vi "Interpret Admin.vi"(8 "error in (no error)":errorcluster, 11 "VISA resource name":refnum<visa-resource-name>) -> (0 "error out":errorcluster, 2 "Trace Admin":T1 {"X at 0" format="%#_3e"; "Y at 0" format="%#_3e"; "X Resolution" format="%#_3e"; "Y Resolution" format="%#_3e"; "X Offset" format="%#_3e"; "Y Offset" format="%#_3e"; "X Step" items=["1-2-5 Range"=1, "Record Range"=3, "Variable Range"=4]; "Y Step" items=["1-2-5 Range"=1, "1-2-4 Range"=2]; "X Divisions" format="%#_3e"; "Y Divisions" format="%#_3e"; "X Unit" items=["None", "Volt", "Ampere", "Ohm", "Watt", "Farad", "Kelvin", "Seconds", "Hours", "Days", "Hertz", "Degree", "Celsius", "Fahrenheit", "Percentage", "dBm 50 Ohm", "dBm 600 Ohm", "dB Volts", "dB Ampere", "dB Watts", "Volt * Ampere Reactive", "Volt * Ampere"]; "Y Unit" items=["None", "Volt", "Ampere", "Ohm", "Watt", "Farad", "Kelvin", "Seconds", "Hours", "Days", "Hertz", "Degree", "Celsius", "Fahrenheit", "Percentage", "dBm 50 Ohm", "dBm 600 Ohm", "dB Volts", "dB Ampere", "dB Watts", "Volt * Ampere Reactive", "Volt * Ampere"]}, 3 "VISA resource name out":refnum<visa-resource-name>)   [LabVIEW 2014, in "Fluke 190 Series II.lvlib"]
doc: "Formats the setup information for a waveform sent by the instrument."
uses:
  Fluke 190 Series II.lvlib
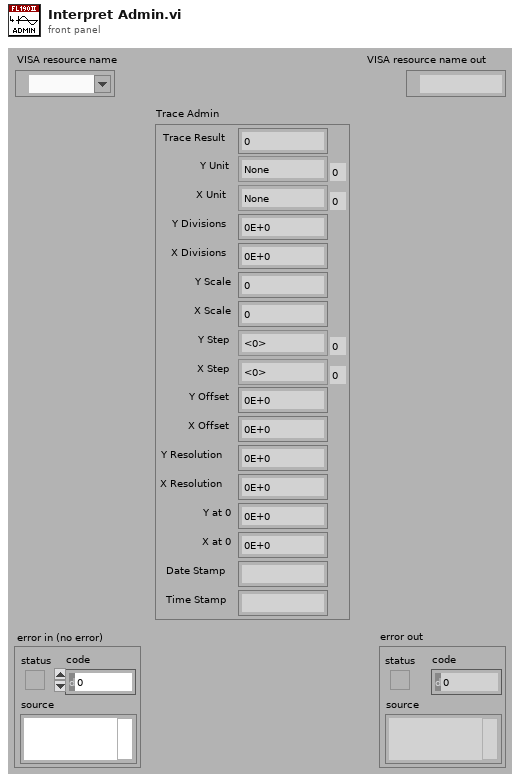
[diagram p1: front panel]
types:
  T1 = cluster{"Trace Result":u8, "Y Unit":u8, "X Unit ":u8, "Y Divisions":u16, "X Divisions":u16, "Y Scale":dbl, "X Scale":dbl, "Y Step":u8, "X Step":u8, "Y Offset":dbl, "X Offset":dbl, "Y Resolution":dbl, "X Resolution":dbl, "Y at 0":dbl, "X at 0":dbl, "Date Stamp":string, "Time Stamp":string}
  T2 = cluster{u8, u8, u8, u16, u16, "Converted Output":dbl, "Converted Output":dbl, u8, u8, "Converted Output":dbl, "Converted Output":dbl, "Converted Output":dbl, "Converted Output":dbl, "Converted Output":dbl, "Converted Output":dbl, "read buffer":string, "read buffer":string}
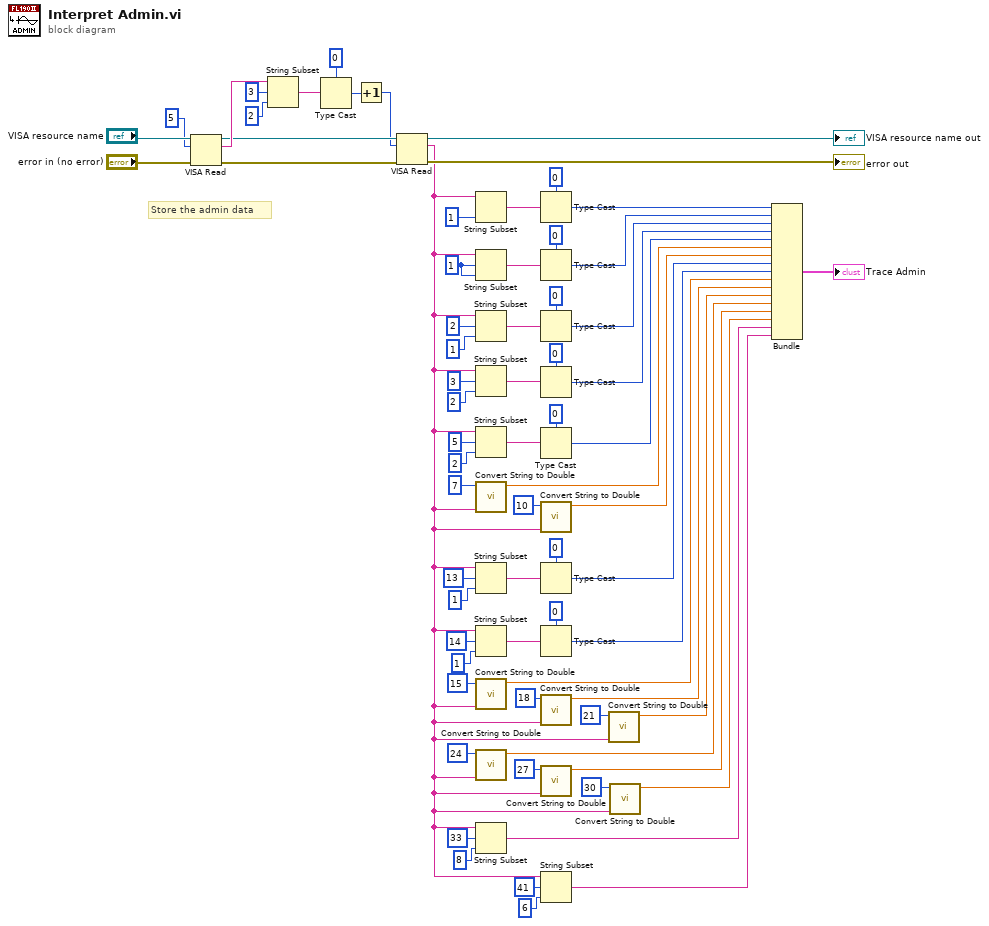
[diagram p0: block diagram]
diagram:
  w51 = 1 ("length (rest)")
  # "Store the admin data"
  n1 = VISA Read(VISA resource name="VISA resource name", byte count=u32 5, error in (no error)="error in (no error)") -> (VISA resource name out=w59:refnum<visa-resource-name>, read buffer=w68:string, error out=w62:errorcluster)  [unwired: 1 out]
  n2 = String Subset(string=w68, offset (0)=3, length (rest)=2 ("length (rest)")) -> (substring=w65:string)
  n3 = Type Cast(type=u16 0, x=w65) -> (*(type *) &x=w63:u16)
  n4 = Increment(x=w63) -> (x+1=w58:u16)
  n5 = VISA Read(VISA resource name=w59, byte count=w58, error in (no error)=w62) -> (VISA resource name out=→"VISA resource name out":refnum<visa-resource-name>, read buffer=w4:string, error out=→"error out":errorcluster)  [unwired: 1 out]
  n6 = String Subset(string=w4, length (rest)=1 ("length (rest)")) -> (substring=w55:string)  [unwired: 1 out]
  n7 = String Subset(string=w4, offset (0)=w51, length (rest)=w51) -> (substring=w52:string)
  n8 = String Subset(string=w4, offset (0)=2, length (rest)=1 ("length (rest)")) -> (substring=w48:string)
  n9 = String Subset(string=w4, offset (0)=3, length (rest)=2 ("length (rest)")) -> (substring=w42:string)
  n10 = String Subset(string=w4, offset (0)=5, length (rest)=2 ("length (rest)")) -> (substring=w39:string)
  n11 = call "Convert String to Double.vi"("Input String"=w4, "String Offset (0)"=7) -> ("Converted Output"=w33:dbl)  [unwired: 1 in, 8 out]
  n12 = String Subset(string=w4, offset (0)=13, length (rest)=1 ("length (rest)")) -> (substring=w29:string)
  n13 = String Subset(string=w4, offset (0)=14, length (rest)=1 ("length (rest)")) -> (substring=w24:string)
  n14 = call "Convert String to Double.vi"("Input String"=w4, "String Offset (0)"=15) -> ("Converted Output"=w19:dbl)  [unwired: 1 in, 8 out]
  n15 = call "Convert String to Double.vi"("Input String"=w4, "String Offset (0)"=24) -> ("Converted Output"=w11:dbl)  [unwired: 1 in, 8 out]
  n16 = String Subset(string=w4, offset (0)=33, length (rest)=8 ("length (rest)")) -> (substring=w6:string)
  n17 = Type Cast(type=u8 0, x=w55) -> (*(type *) &x=w54:u8)
  n18 = Type Cast(type=u8 0, x=w52) -> (*(type *) &x=w50:u8)
  n19 = Type Cast(type=u8 0, x=w48) -> (*(type *) &x=w45:u8)
  n20 = Type Cast(type=u16 0, x=w42) -> (*(type *) &x=w40:u16)
  n21 = Type Cast(type=u16 0, x=w39) -> (*(type *) &x=w35:u16)
  n22 = call "Convert String to Double.vi"("Input String"=w4, "String Offset (0)"=10) -> ("Converted Output"=w31:dbl)  [unwired: 1 in, 8 out]
  n23 = Type Cast(type=u8 0, x=w29) -> (*(type *) &x=w26:u8)
  n24 = Type Cast(type=u8 0, x=w24) -> (*(type *) &x=w21:u8)
  n25 = call "Convert String to Double.vi"("Input String"=w4, "String Offset (0)"=18) -> ("Converted Output"=w17:dbl)  [unwired: 1 in, 8 out]
  n26 = call "Convert String to Double.vi"("Input String"=w4, "String Offset (0)"=27) -> ("Converted Output"=w10:dbl)  [unwired: 1 in, 8 out]
  n27 = String Subset(string=w4, offset (0)=41, length (rest)=6 ("length (rest)")) -> (substring=w5:string)
  n28 = call "Convert String to Double.vi"("Input String"=w4, "String Offset (0)"=21) -> ("Converted Output"=w15:dbl)  [unwired: 1 in, 8 out]
  n29 = call "Convert String to Double.vi"("Input String"=w4, "String Offset (0)"=30) -> ("Converted Output"=w9:dbl)  [unwired: 1 in, 8 out]
  n30 = Bundle(w54, w50, w45, w40, w35, "Converted Output"=w33, "Converted Output"=w31, w26, w21, "Converted Output"=w19, "Converted Output"=w17, "Converted Output"=w15, "Converted Output"=w11, "Converted Output"=w10, "Converted Output"=w9, "read buffer"=w6, "read buffer"=w5) -> (→"Trace Admin":T2)  [unwired: 1 out]
